vi "PH_Beamline_Chief.get Section Status Tagname.vi"(1 "Beamline Section":T1) -> (0 "Section Status Tagname":string)   [LabVIEW 2014, in "PH_Beamline_Chief.lvlib"]
doc: "This VI concatenates a Tagname out of strict type def enum controls. It keeps also the information whether the Tag is existing (if not, N/A is given out as name)."
uses:
  PH_Beamline_Chief.lvlib
  PH_Beamline_Chief.Section.ctl
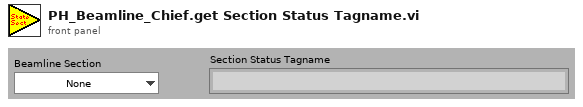
[diagram p1: front panel]
types:
  T1 = typedef "PH_Beamline_Chief.lvlib/PH_Beamline_Chief.Section.ctl" = enum16{"None", "YLF", "fs", "fs-YLF", "ns", "PA-Input", "PA-Undelay", "PA-Delay", "PA-before-Bypass", "PA", "PA-Bypass", "PA-Exit", "PA-LL", "LL", "PA-MA", "MA-Exit", "MA-Z6", "Z6", "MA-LB", "LB-TB2", "LB-TB3"}
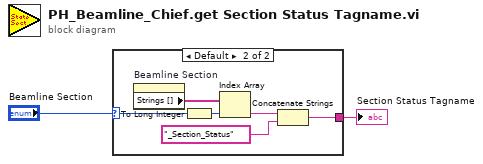
[diagram p0: block diagram]
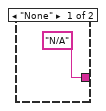
[diagram p2: hidden frame]
diagram:
  n1 = case shown="Default" "Beamline Section" {
    selector: "Beamline Section" -> [_ w7]
    tunnel: ["N/A" w9] -> w2
    frame "None" {
    }
    frame Default {
      n2 = property on="Beamline Section" class="Enum (strict)"() -> ("Strings []"=w8:string[])  [unwired: 2 in, 2 out]
      n3 = To Long Integer(number=w7) -> (32bit integer=w6:i32)
      n4 = Index Array(array=w8, index=w6) -> (element=w5:string)
      n5 = Concatenate Strings(w5, "_Section_Status" ("string")) -> (w9:string)
    }
  }
  "Section Status Tagname" <- w2
